vi "ChangeExtension.vi"(6 "error in (no error)":errorcluster, 7 "extension":string="dat", 8 "file in":string="E:\\users\\noort\\data\\270404\\_001.log", 9 "Path in":path=path "") -> (0 "error out":errorcluster, 1 "Tracenr":string, 2 "file out":string=".dat", 3 "Path out":path=path ".dat", 4 "Tracenr":i32)   [LabVIEW 2018]
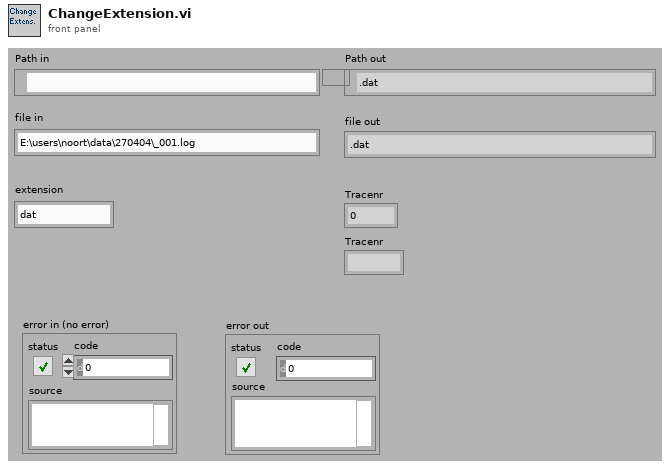
[diagram p1: front panel]
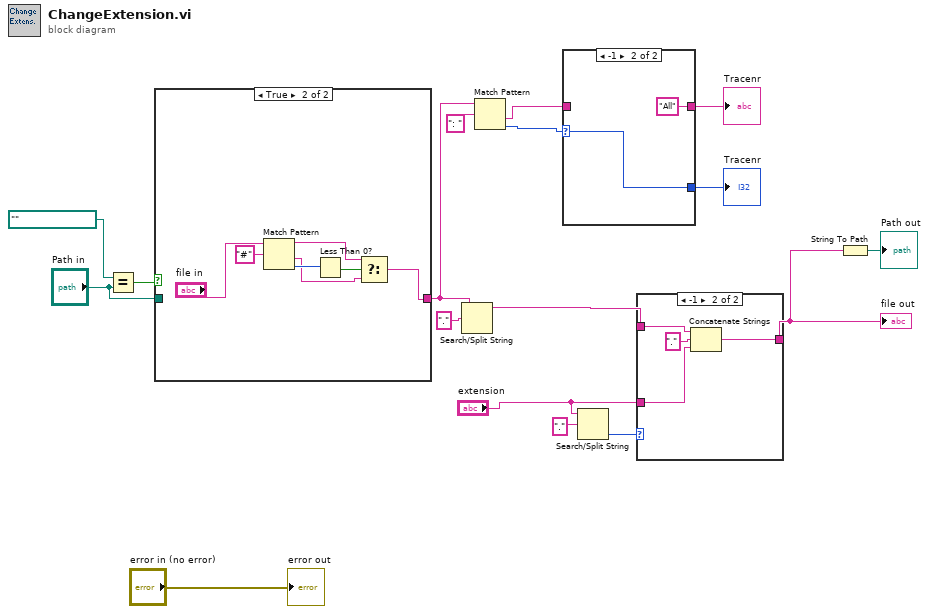
[diagram p0: block diagram]
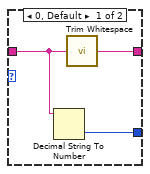
[diagram p2: hidden frame]
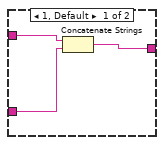
[diagram p3: hidden frame]
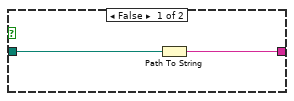
[diagram p4: hidden frame]
diagram:
  n1 = Equal?(x=path "" ("Path in"), y="Path in") -> (x = y?=w14:bool)
  n2 = case shown="True" w14 {
    tunnel: [w18 w20] -> w5
    tunnel: "Path in" -> [w19 _]
    frame False {
      n3 = Path To String(path=w19) -> (string=w18:string)
    }
    frame True {
      n4 = Match Pattern(string="file in", regular expression="#") -> (before substring=w21:string, after substring=w22:string, offset past match=w24:i32)  [unwired: 1 in, 1 out]
      n5 = Less Than 0?(x=w24) -> (x < 0?=w23:bool)
      n6 = Select(t=w21, s=w23, f=w22) -> (s? t:f=w20:string)
    }
  }
  n7 = Search/Split String(string=w5, search string/char (-)=".") -> (substring before match=w16:string)  [unwired: 1 in, 2 out]
  n8 = Match Pattern(string=w5, regular expression=": " ("search string/char (-)")) -> (after substring=w3:string, offset past match=w2:i32)  [unwired: 1 in, 2 out]
  n9 = case shown="-1" w2 {
    selector: w2 -> [_ w31]
    tunnel: [w29 w31] -> w7
    tunnel: [w28 "All" ("trimmed string")] -> w6
    tunnel: w3 -> [w27 _]
    frame 0, Default {
      n10 = Decimal String To Number(string=w27) -> (number=w29:i32)  [unwired: 2 in, 1 out]
      n11 = call <vilib>:"Trim Whitespace.vi"("string"=w27) -> ("trimmed string"=w28:string)  [unwired: 1 in]
    }
    frame -1 {
    }
  }
  "Tracenr" <- w7
  "Tracenr" <- w6
  n12 = Search/Split String(string="extension", search string/char (-)=".") -> (offset of match=w9:i32)  [unwired: 1 in, 2 out]
  n13 = case shown="-1" w9 {
    tunnel: w16 -> [w34 w37]
    tunnel: [w33 w36] -> w13
    tunnel: "extension" -> [w32 w35]
    frame 1, Default {
      n14 = Concatenate Strings(w34, w32) -> (w33:string)
    }
    frame -1 {
      n15 = Concatenate Strings(w37, "." ("Substring"), w35) -> (w36:string)
    }
  }
  "file out" <- w13
  n16 = String To Path(string=w13) -> (path=→"Path out":path)
  "error out" <- "error in (no error)"
